vi "PosNotifyGen.vi"() -> (0 "PositionRef":cluster{"X":dbl, "Y":dbl}, 1 "PosNotifyRef":refnum<notifier>)   [LabVIEW 2012]
panel:
  in  "Position":cluster{"X":dbl, "Y":dbl}
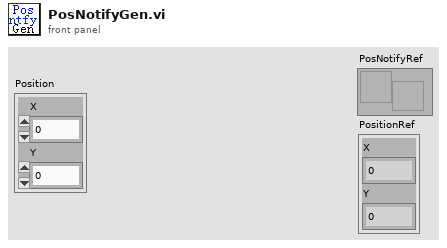
[diagram p1: front panel]
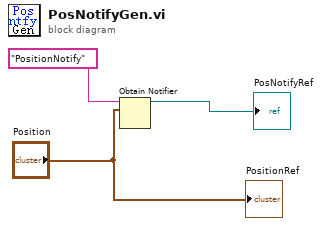
[diagram p0: block diagram]
diagram:
  n1 = Obtain Notifier(name (unnamed)="PositionNotify" ("名称（未命名）"), notification data type="Position") -> (notifier out=→"PosNotifyRef":refnum<notifier>)  [unwired: 2 in, 2 out]
  "PositionRef" <- "Position"
